vi "CRYASIOForceInitialize.vi"(8 "Sampling Rate":u32, 9 "Driver Name":string, 11 "error in (no error)":errorcluster) -> (0 "bResult":bool, 3 "error out":errorcluster)   [LabVIEW 2013]
uses:
  CRYASIO Global.vi
  CRY_ASIO.dll
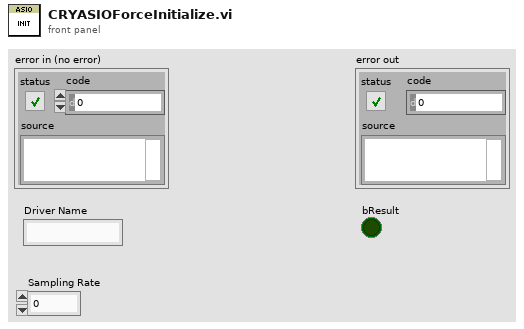
[diagram p1: front panel]
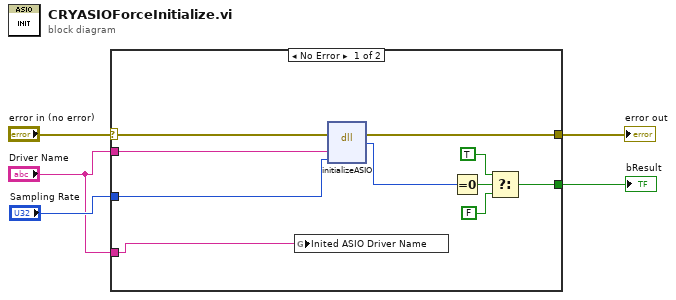
[diagram p0: block diagram]
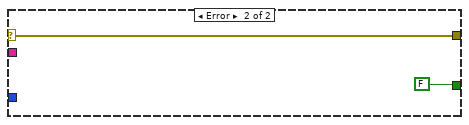
[diagram p2: hidden frame]
diagram:
  n1 = case shown="No Error" "error in (no error)" {
    selector: "error in (no error)" -> [w15 w17]
    tunnel: [w14 w17] -> w4
    tunnel: "Driver Name" -> [w11 _]
    tunnel: "Sampling Rate" -> [w13 _]
    tunnel: [w12 FALSE] -> w2
    tunnel: "Driver Name" -> [w6 _]
    frame No Error {
      n2 = global write "CRYASIO Global.vi" "Inited ASIO Driver Name"(w6) -> ()
      n3 = dll-call lib="D:/LabView_Project/CRY6181/CRY_ASIO.dll" fn="initializeASIO"(error in=w15, "arg1"=w11, "arg2"=w13) -> (error out=w14:errorcluster, "return type"=w9:i32)  [unwired: 4 in, 1 out]
      n4 = Equal To 0?(x=w9) -> (x = 0?=w10:bool)
      n5 = Select(t=TRUE, s=w10, f=FALSE) -> (s? t:f=w12:bool)
    }
    frame Error {
    }
  }
  "error out" <- w4
  "bResult" <- w2
